vi "_API_BINANCE_GET_Klines_CandlestickData.vi"(0 "BinanceAPI in":refnum<class "BinanceAPI_.lvclass">, 5 "Klines/Candlestick_PARAMS":T1={"symbol"="", "interval"=enum."3m", "startTime"=0, "endTime"=0, "limit"=0}, 11 "error in (no error)":errorcluster) -> (4 "BinanceAPI out":refnum<class "BinanceAPI_.lvclass">, 6 "Klines":dbl[][](array[numeric]) format="%#.6g", 14 "Dane":string, 15 "error out":errorcluster)   [LabVIEW 2022 SP3, in "BinanceAPI_.lvclass"]
doc: "https://binance-docs.github.io/apidocs/spot/en/#kline-candlestick-data"
uses:
  BinanceAPI_.lvclass
  BinanceAPI_.lvclass/BinanceAPI_.ctl
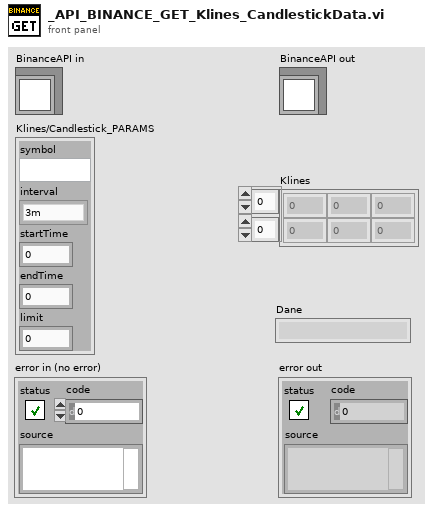
[diagram p1: front panel]
types:
  T1 = cluster{"symbol":string, "interval":enum16{"NaN", "1m", "3m", "5m", "15m", "30m", "1h", "2h", "4h", "6h", "8h", "12h", "1d", "3d", "1w", "1M"}, "startTime":i32, "endTime":i32, "limit":i16}
  T2 = enum16{"NaN", "1m", "3m", "5m", "15m", "30m", "1h", "2h", "4h", "6h", "8h", "12h", "1d", "3d", "1w", "1M"}
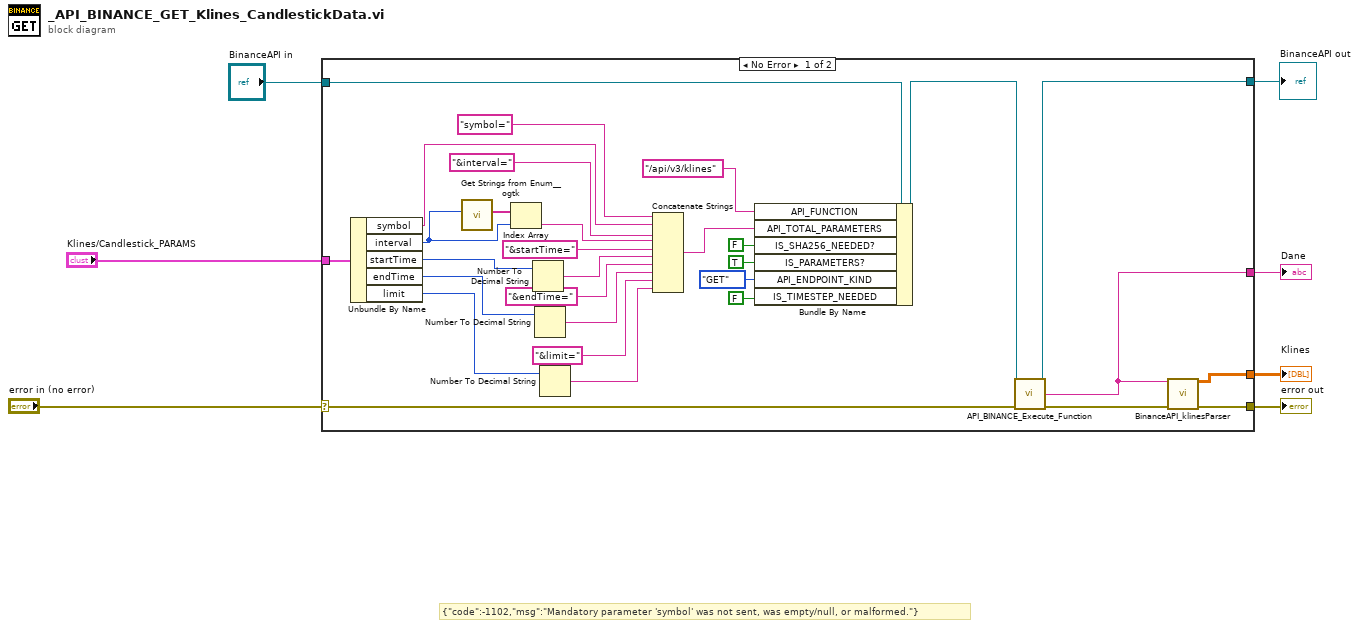
[diagram p0: block diagram]
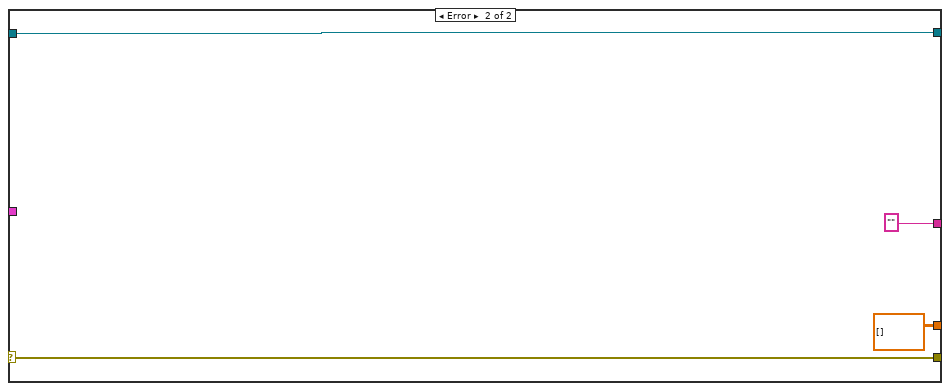
[diagram p2: hidden frame]
diagram:
  # "{\"code\":-1102,\"msg\":\"Mandatory parameter 'symbol' was not sent, was empty/null, or malformed.\"}"
  n1 = case shown="No Error" "error in (no error)" {
    selector: "error in (no error)" -> [w13 w41]
    tunnel: [w10 w41] -> w6
    tunnel: [w14 w40] -> w1
    tunnel: "BinanceAPI in" -> [w27 w40]
    tunnel: "Klines/Candlestick_PARAMS" -> [w33 _]
    tunnel: [w9 "" ("Dane")] -> w4
    tunnel: [w8 dbl[][] [] ("Klines")] -> w3
    frame No Error {
      n2 = Unbundle By Name(w33) -> ("symbol"=w17:string, "interval"=w19:T2, "startTime"=w30:i32, "endTime"=w29:i32, "limit"=w28:i16)
      n3 = call <userlib>:"Get Strings from Enum__ogtk.vi"("Enum"=w19) -> ("Enum Strings"=w20:string[])  [unwired: 7 in, 3 out]
      n4 = Index Array(array=w20, index=w19) -> (element=w16:string)
      n5 = Number To Decimal String(number=w30) -> (decimal integer string=w25:string)  [unwired: 1 in]
      n6 = Number To Decimal String(number=w29) -> (decimal integer string=w23:string)  [unwired: 1 in]
      n7 = Number To Decimal String(number=w28) -> (decimal integer string=w21:string)  [unwired: 1 in]
      n8 = Concatenate Strings("symbol=" ("API_FUNCTION 2"), w17, "&interval=" ("API_FUNCTION 2"), w16, "&startTime=" ("API_FUNCTION 2"), w25, "&endTime=" ("API_FUNCTION 2"), w23, "&limit=" ("API_FUNCTION 2"), w21) -> (w34:string)
      n9 = Bundle By Name(cluster=w27, "API_FUNCTION"="/api/v3/klines", "API_TOTAL_PARAMETERS"=w34, "IS_SHA256_NEEDED?"=FALSE, "IS_PARAMETERS?"=TRUE, "API_ENDPOINT_KIND"=enum16{"POST", "DELETE", "GET", "PUT"}."GET", "IS_TIMESTEP_NEEDED"=FALSE) -> (w15:refnum<class "BinanceAPI_.lvclass">)
      n10 = call "API_BINANCE_Execute_Function.vi"("BinanceAPI in"=w15, "error in (no error)"=w13) -> ("BinanceAPI out"=w14:refnum<class "BinanceAPI_.lvclass">, "Body"=w9:string, "error out"=w11:errorcluster)  [unwired: 9 in, 2 out]
      n11 = call "BinanceAPI_klinesParser.vi"("String"=w9, "error in (no error)"=w11) -> ("Klines"=w8:dbl[][], "error out"=w10:errorcluster)  [unwired: 12 in]
    }
    frame Error {
    }
  }
  "error out" <- w6
  "Dane" <- w4
  "Klines" <- w3
  "BinanceAPI out" <- w1
